vi "Lab Panel V5.40.vi"() -> ()   [LabVIEW 2017] (continued)
                    n2206 = Multiply(x=w3869, y=w3863) -> (x*y=w3856:dbl)
                    n2207 = Multiply(x=w3868, y=w3862) -> (x*y=w3854:dbl)
                    n2208 = Multiply(x=w3867, y=w3861) -> (x*y=w3853:dbl)
                    n2209 = Multiply(x=w3866, y=w3860) -> (x*y=w3852:dbl)
                    n2210 = local read "SIG LAB02-1"() -> (w3859:T2)
                    n2211 = local read "SIG LAB02-2"() -> (w3855:T2)
                    n2212 = Bundle By Name(cluster=w3859, "AMPS"=w3858, "VOLTS"=w3857, "PF"=w3856) -> (w3851:T2)
                    n2213 = Bundle By Name(cluster=w3855, "AMPS"=w3854, "VOLTS"=w3853, "PF"=w3852) -> (w3850:T2)
                    n2214 = global write "Global display 1.vi" "SIG LAB02-1"(w3851) -> ()
                    n2215 = local write "SIG LAB02-2"(w3850) -> ()
                    n2216 = global write "Global display 1.vi" "SIG LAB02-2"(w3850) -> ()
                    n2217 = local write "SIG LAB02-1"(w3851) -> ()
                  }
                  frame #4 {
                    n2218 = Unbundle By Name(w3903) -> ("OFF amps"=w3899:dbl, "VOLTS"=w3898:dbl, "PF"=w3897:dbl, "OFF amps"=w3896:dbl, "VOLTS"=w3895:dbl, "PF"=w3894:dbl)
                    n2219 = case shown="True" w3902 {
                      tunnel: [w3904 w3905] -> w3900
                      tunnel: w3901 -> [_ w3905]
                      frame False {
                        n2220 = local read "CAL LAB03"() -> (w3904:T15)
                      }
                      frame True {
                      }
                    }
                    n2221 = Unbundle By Name(w3900) -> ("1  (A) cal"=w3893:dbl, "1 (V) cal"=w3892:dbl, "1 (PF) cal"=w3891:dbl, "2 (A) cal"=w3890:dbl, "2 (V) cal"=w3889:dbl, "2 (PF) cal"=w3888:dbl)  [unwired: 4 out]
                    n2222 = Multiply(x=w3899, y=w3893) -> (x*y=w3886:dbl)
                    n2223 = Multiply(x=w3898, y=w3892) -> (x*y=w3880:dbl)
                    n2224 = Multiply(x=w3897, y=w3891) -> (x*y=w3885:dbl)
                    n2225 = Multiply(x=w3896, y=w3890) -> (x*y=w3883:dbl)
                    n2226 = Multiply(x=w3895, y=w3889) -> (x*y=w3882:dbl)
                    n2227 = Multiply(x=w3894, y=w3888) -> (x*y=w3881:dbl)
                    n2228 = local read "SIG LAB03-1"() -> (w3887:T2)
                    n2229 = local read "SIG LAB03-2"() -> (w3884:T2)
                    n2230 = Bundle By Name(cluster=w3887, "AMPS"=w3886, "VOLTS"=w3880, "PF"=w3885) -> (w3879:T2)
                    n2231 = Bundle By Name(cluster=w3884, "AMPS"=w3883, "VOLTS"=w3882, "PF"=w3881) -> (w3878:T2)
                    n2232 = global write "Global display 1.vi" "SIG LAB03-1"(w3879) -> ()
                    n2233 = global write "Global display 1.vi" "SIG LAB03-2"(w3878) -> ()
                    n2234 = local write "SIG LAB03-2"(w3878) -> ()
                    n2235 = local write "SIG LAB03-1"(w3879) -> ()
                  }
                  frame #5 {
                    n2236 = case shown="False" w3930 {
                      tunnel: [w3932 w3933] -> w3928
                      tunnel: w3929 -> [_ w3933]
                      frame False {
                        n2237 = local read "CAL LAB04"() -> (w3932:T15)
                      }
                      frame True {
                      }
                    }
                    n2238 = Unbundle By Name(w3931) -> ("OFF amps"=w3927:dbl, "VOLTS"=w3926:dbl, "PF"=w3925:dbl, "OFF amps"=w3924:dbl, "VOLTS"=w3923:dbl, "PF"=w3922:dbl)
                    n2239 = Unbundle By Name(w3928) -> ("1  (A) cal"=w3921:dbl, "1 (V) cal"=w3920:dbl, "1 (PF) cal"=w3919:dbl, "2 (A) cal"=w3918:dbl, "2 (V) cal"=w3917:dbl, "2 (PF) cal"=w3916:dbl)  [unwired: 4 out]
                    n2240 = Multiply(x=w3927, y=w3921) -> (x*y=w3914:dbl)
                    n2241 = Multiply(x=w3926, y=w3920) -> (x*y=w3913:dbl)
                    n2242 = Multiply(x=w3925, y=w3919) -> (x*y=w3912:dbl)
                    n2243 = Multiply(x=w3924, y=w3918) -> (x*y=w3910:dbl)
                    n2244 = Multiply(x=w3923, y=w3917) -> (x*y=w3909:dbl)
                    n2245 = Multiply(x=w3922, y=w3916) -> (x*y=w3908:dbl)
                    n2246 = local read "SIG LAB04-1"() -> (w3915:T2)
                    n2247 = local read "SIG LAB04-2"() -> (w3911:T2)
                    n2248 = Bundle By Name(cluster=w3915, "AMPS"=w3914, "VOLTS"=w3913, "PF"=w3912) -> (w3907:T2)
                    n2249 = Bundle By Name(cluster=w3911, "AMPS"=w3910, "VOLTS"=w3909, "PF"=w3908) -> (w3906:T2)
                    n2250 = global write "Global display 1.vi" "SIG LAB04-2"(w3906) -> ()
                    n2251 = global write "Global display 1.vi" "SIG LAB04-1"(w3907) -> ()
                    n2252 = local write "SIG LAB04-2"(w3906) -> ()
                    n2253 = local write "SIG LAB04-1"(w3907) -> ()
                  }
                  frame #6 {
                    n2254 = Unbundle By Name(w3959) -> ("OFF amps"=w3955:dbl, "VOLTS"=w3936:dbl, "PF"=w3954:dbl, "OFF amps"=w3953:dbl, "VOLTS"=w3952:dbl, "PF"=w3951:dbl)
                    n2255 = case shown="False" w3958 {
                      tunnel: [w3960 w3961] -> w3956
                      tunnel: w3957 -> [_ w3961]
                      frame False {
                        n2256 = local read "CAL LAB05"() -> (w3960:T15)
                      }
                      frame True {
                      }
                    }
                    n2257 = Unbundle By Name(w3956) -> ("1  (A) cal"=w3950:dbl, "1 (V) cal"=w3949:dbl, "1 (PF) cal"=w3948:dbl, "2 (A) cal"=w3947:dbl, "2 (V) cal"=w3946:dbl, "2 (PF) cal"=w3945:dbl)  [unwired: 4 out]
                    n2258 = Multiply(x=w3955, y=w3950) -> (x*y=w3943:dbl)
                    n2259 = Multiply(x=w3936, y=w3949) -> (x*y=w3942:dbl)
                    n2260 = Multiply(x=w3954, y=w3948) -> (x*y=w3941:dbl)
                    n2261 = Multiply(x=w3953, y=w3947) -> (x*y=w3939:dbl)
                    n2262 = Multiply(x=w3952, y=w3946) -> (x*y=w3938:dbl)
                    n2263 = Multiply(x=w3951, y=w3945) -> (x*y=w3937:dbl)
                    n2264 = local read "SIG LAB05-1"() -> (w3944:T2)
                    n2265 = local read "SIG LAB05-2"() -> (w3940:T2)
                    n2266 = Bundle By Name(cluster=w3944, "AMPS"=w3943, "VOLTS"=w3942, "PF"=w3941) -> (w3935:T2)
                    n2267 = Bundle By Name(cluster=w3940, "AMPS"=w3939, "VOLTS"=w3938, "PF"=w3937) -> (w3934:T2)
                    n2268 = global write "Global display 1.vi" "SIG LAB05-1"(w3935) -> ()
                    n2269 = global write "Global display 1.vi" "SIG LAB05-2"(w3934) -> ()
                    n2270 = local write "SIG LAB05-2"(w3934) -> ()
                    n2271 = local write "SIG LAB05-1"(w3935) -> ()
                  }
                  frame #7 {
                    n2272 = case shown="False" w3962 {
                      tunnel: w3964 -> [w3969 _]
                      tunnel: w3963 -> [w3968 _]
                      frame False {
                        # "update ambient referance temperature"
                        n2273 = case shown="True" w3969 {
                          tunnel: [w3971 100.0] -> w3970
                          frame False {
                            n2274 = local read "TEMP REF cal"() -> (w3971:dbl)
                          }
                          frame True {
                          }
                        }
                        n2275 = disable-structure shown="Disabled" {
                          frame Disabled {
                            n2276 = local read "Temp read loop"() -> ()  [unwired: 1 out]
                          }
                          frame Enabled {
                          }
                        }
                        n2277 = Multiply(x=w3970, y=w3968) -> (x*y=w3967:dbl)
                        n2278 = Subtract(x=w3967, y=272) -> (x-y=w3965:dbl)
                        "Amb Tp" <- w3965
                        n2279 = local write "Ref deg C"(w3965) -> ()
                        "deg C (volts)" <- w3968
                      }
                      frame True {
                      }
                    }
                  }
                }
              }
            }
          }
          frame #14 {
            # "save test data to file during testing"
            n2280 = local read "on loops"() -> (w3992:dbl)
            n2281 = Get Date/Time In Seconds() -> (seconds since 1Jan1904=w3973:timestamp)
            "File Time Stamp" <- w3973
            n2282 = local read "jig cycle"() -> (w3989:dbl)
            n2283 = Format Date/Time String(time format string (%c)="%H:%M%:%S", seconds (now)=w3973) -> (date/time string=w3977:string)  [unwired: 1 in]
            n2284 = Add(x=w3992, y=4) -> (x+y=w3990:dbl)
            n2285 = Build Array(w3977) -> (w3976:string[])
            n2286 = Equal?(x=w3989, y=3) -> (x = y?=w3975:bool)
            n2287 = Equal?(x=w3989, y=w3990) -> (x = y?=w3974:bool)
            n2288 = stacked-sequence {
              tunnel: w3988 -> [w3998 _ _ _ _ _ _ _ _ _]
              tunnel: w3987 -> [_ w4074 _ _ _ _ _ _ _ _]
              tunnel: w3986 -> [_ _ w4154 _ _ _ _ _ _ _]
              tunnel: w3985 -> [_ _ _ w4234 _ _ _ _ _ _]
              tunnel: w3984 -> [_ _ _ _ w4314 _ _ _ _ _]
              tunnel: w3983 -> [_ _ _ _ _ w4394 _ _ _ _]
              tunnel: w3982 -> [_ _ _ _ _ _ w4474 _ _ _]
              tunnel: w3981 -> [_ _ _ _ _ _ _ w4554 _ _]
              tunnel: w3980 -> [_ _ _ _ _ _ _ _ w4634 _]
              tunnel: w3979 -> [_ _ _ _ _ _ _ _ _ w4714]
              tunnel: w3976 -> [w3997 w4078 w4158 w4238 w4318 w4398 w4478 w4558 w4638 w4718]
              tunnel: w3975 -> [w3996 w4077 w4157 w4237 w4317 w4397 w4477 w4557 w4637 w4717]
              tunnel: w3974 -> [w3995 w4076 w4156 w4236 w4316 w4396 w4476 w4556 w4636 w4716]
              tunnel: w3973 -> [w3994 w4075 w4155 w4235 w4315 w4395 w4475 w4555 w4635 w4715]
              frame #0 {
                n2289 = case shown="True" w3998 {
                  tunnel: w3997 -> [_ w4003]
                  tunnel: w3996 -> [_ w4002]
                  tunnel: w3995 -> [_ w4000]
                  tunnel: w3994 -> [_ w3999]
                  frame False {
                  }
                  frame True {
                    n2290 = local read "SIG LAB01-1"() -> (w4005:T2)
                    n2291 = local read "ON L01-1"() -> (w4001:cluster{"amps":dbl, "volts":dbl, "pf":dbl})
                    n2292 = local read "DISP LAB01-1"() -> (w4004:T4)
                    n2293 = Unbundle(w4005) -> ("AMPS"=w4011:dbl, "VOLTS"=w4009:dbl, "PF"=w4008:dbl, "Tmp Live"=w4007:dbl, "Tmp Neut"=w4010:dbl)
                    n2294 = Unbundle(w4004) -> ("CYCLE"=w4006:dbl)  [unwired: 2 out]
                    n2295 = stacked-sequence {
                      tunnel: w4011 -> [w4015 w4034]
                      tunnel: w4010 -> [_ w4033]
                      tunnel: w4009 -> [w4014 w4032]
                      tunnel: w4008 -> [w4013 w4031]
                      tunnel: w4007 -> [_ w4030]
                      tunnel: w4006 -> [_ w4029]
                      tunnel: w4003 -> [_ w4028]
                      tunnel: w4002 -> [w4016 _]
                      tunnel: w4001 -> [w4012 w4026]
                      tunnel: w4000 -> [_ w4027]
                      tunnel: w3999 -> [_ w4022]
                      frame #0 {
                        n2296 = case shown="True" w4016 {
                          tunnel: w4015 -> [_ w4021]
                          tunnel: w4014 -> [_ w4020]
                          tunnel: w4013 -> [_ w4019]
                          tunnel: w4012 -> [_ w4017]
                          frame False {
                          }
                          frame True {
                            n2297 = Bundle(cluster=w4017, "amps"=w4021, "volts"=w4020, "pf"=w4019) -> (w4018:cluster{"amps":dbl, "volts":dbl, "pf":dbl})
                            n2298 = local write "ON L01-1"(w4018) -> ()
                          }
                        }
                      }
                      frame #1 {
                        n2299 = Unbundle(w4026) -> ("amps"=w4025:dbl, "volts"=w4024:dbl, "pf"=w4023:dbl)
                        n2300 = case shown="True" w4027 {
                          tunnel: w4034 -> [_ w4035]
                          tunnel: w4033 -> [_ w4073]
                          tunnel: w4032 -> [_ _]
                          tunnel: w4031 -> [_ _]
                          tunnel: w4030 -> [_ w4072]
                          tunnel: w4029 -> [_ w4071]
                          tunnel: w4028 -> [_ w4039]
                          tunnel: w4025 -> [_ w4036]
                          tunnel: w4024 -> [_ w4068]
                          tunnel: w4023 -> [_ w4067]
                          tunnel: w4022 -> [_ w4037]
                          frame False {
                          }
                          frame True {
                            n2301 = local read "TDMS LAB01-1"() -> (w4070:refnum<k34>)
                            n2302 = Build Array(w4068) -> (w4064:dbl[])
                            n2303 = Build Array(w4067) -> (w4063:dbl[])
                            n2304 = Build Array(w4072) -> (w4062:dbl[])
                            n2305 = Build Array(w4073) -> (w4061:dbl[])
                            n2306 = Build Array(w4036) -> (w4066:dbl[])
                            n2307 = Build Array(w4035) -> (w4065:dbl[])
                            n2308 = Build Array(w4071) -> (w4060:dbl[])
                            n2309 = Build Array("AMPS ON", "AMPS OFF", "VOLTS", "PF", "TEMP Live", "TEMP Neut", "CYCLE") -> (w4044:string[])
                            n2310 = Bundle By Name("Y"=w4066, "t0"=w4037) -> (w4059:waveform(dbl))  [unwired: 1 in]
                            n2311 = Bundle By Name("Y"=w4065, "t0"=w4037) -> (w4058:waveform(dbl))  [unwired: 1 in]
                            n2312 = Bundle By Name("Y"=w4064, "t0"=w4037) -> (w4057:waveform(dbl))  [unwired: 1 in]
                            n2313 = Bundle By Name("Y"=w4063, "t0"=w4037) -> (w4056:waveform(dbl))  [unwired: 1 in]
                            n2314 = Bundle By Name("Y"=w4062, "t0"=w4037) -> (w4055:waveform(dbl))  [unwired: 1 in]
                            n2315 = Bundle By Name("Y"=w4061, "t0"=w4037) -> (w4054:waveform(dbl))  [unwired: 1 in]
                            n2316 = Bundle By Name("Y"=w4060, "t0"=w4037) -> (w4053:waveform(dbl))  [unwired: 1 in]
                            n2317 = Build Array(w4059, w4058, w4057, w4056, w4055, w4054, w4053) -> (w4052:waveform(dbl)[])
                            n2318 = TDMS Write(0:w4070, 5:"TEST VALUES", 7:w4044, 9:w4052) -> (4:w4043:refnum<k34>, 6:w4042:string, 15:w4041:errorcluster)  [unwired: 2 in, 1 out]
                            n2319 = TDMS Write(0:w4043, 5:w4042, 7:"TIME", 9:w4039, 11:w4041) -> (15:w4038:errorcluster)  [unwired: 1 in, 3 out]
                            n2320 = local write "data file error"(w4038) -> ()
                          }
                        }
                      }
                    }
                  }
                }
              }
              frame #1 {
                n2321 = case shown="True" w4074 {
                  tunnel: w4078 -> [_ w4083]
                  tunnel: w4077 -> [_ w4082]
                  tunnel: w4076 -> [_ w4080]
                  tunnel: w4075 -> [_ w4079]
                  frame False {
                  }
                  frame True {
                    n2322 = local read "DISP LAB01-2"() -> (w4084:T4)
                    n2323 = local read "SIG LAB01-2"() -> (w4085:T2)
                    n2324 = local read "ON L01-2"() -> (w4081:cluster{"amps":dbl, "volts":dbl, "pf":dbl})
                    n2325 = Unbundle(w4085) -> ("AMPS"=w4091:dbl, "VOLTS"=w4089:dbl, "PF"=w4088:dbl, "Tmp Live"=w4087:dbl, "Tmp Neut"=w4090:dbl)
                    n2326 = Unbundle(w4084) -> ("CYCLE"=w4086:dbl)  [unwired: 2 out]
                    n2327 = stacked-sequence {
                      tunnel: w4091 -> [w4095 w4114]
                      tunnel: w4090 -> [_ w4113]
                      tunnel: w4089 -> [w4094 w4112]
                      tunnel: w4088 -> [w4093 w4111]
                      tunnel: w4087 -> [_ w4110]
                      tunnel: w4086 -> [_ w4109]
                      tunnel: w4083 -> [_ w4108]
                      tunnel: w4082 -> [w4096 _]
                      tunnel: w4081 -> [w4092 w4106]
                      tunnel: w4080 -> [_ w4107]
                      tunnel: w4079 -> [_ w4102]
                      frame #0 {
                        n2328 = case shown="True" w4096 {
                          tunnel: w4095 -> [_ w4101]
                          tunnel: w4094 -> [_ w4100]
                          tunnel: w4093 -> [_ w4099]
                          tunnel: w4092 -> [_ w4097]
                          frame False {
                          }
                          frame True {
                            n2329 = Bundle(cluster=w4097, "amps"=w4101, "volts"=w4100, "pf"=w4099) -> (w4098:cluster{"amps":dbl, "volts":dbl, "pf":dbl})
                            n2330 = local write "ON L01-2"(w4098) -> ()
                          }
                        }
                      }
                      frame #1 {
                        n2331 = Unbundle(w4106) -> ("amps"=w4105:dbl, "volts"=w4104:dbl, "pf"=w4103:dbl)
                        n2332 = case shown="True" w4107 {
                          tunnel: w4114 -> [_ w4146]
                          tunnel: w4113 -> [_ w4153]
                          tunnel: w4112 -> [_ _]
                          tunnel: w4111 -> [_ _]
                          tunnel: w4110 -> [_ w4152]
                          tunnel: w4109 -> [_ w4151]
                          tunnel: w4108 -> [_ w4116]
                          tunnel: w4105 -> [_ w4148]
                          tunnel: w4104 -> [_ w4147]
                          tunnel: w4103 -> [_ w4145]
                          tunnel: w4102 -> [_ w4137]
                          frame False {
                          }
                          frame True {
                            n2333 = local read "TDMS LAB01-2"() -> (w4150:refnum<k34>)
                            n2334 = Build Array(w4147) -> (w4142:dbl[])
                            n2335 = Build Array(w4145) -> (w4141:dbl[])
                            n2336 = Build Array(w4152) -> (w4140:dbl[])
                            n2337 = Build Array(w4153) -> (w4139:dbl[])
                            n2338 = Build Array(w4148) -> (w4144:dbl[])
                            n2339 = Build Array(w4146) -> (w4143:dbl[])
                            n2340 = Build Array(w4151) -> (w4138:dbl[])
                            n2341 = Build Array("AMPS ON", "AMPS OFF", "VOLTS", "PF", "TEMP Live", "TEMP Neut", "CYCLE") -> (w4121:string[])
                            n2342 = Bundle By Name("Y"=w4144, "t0"=w4137) -> (w4136:waveform(dbl))  [unwired: 1 in]
                            n2343 = Bundle By Name("Y"=w4143, "t0"=w4137) -> (w4135:waveform(dbl))  [unwired: 1 in]
                            n2344 = Bundle By Name("Y"=w4142, "t0"=w4137) -> (w4134:waveform(dbl))  [unwired: 1 in]
                            n2345 = Bundle By Name("Y"=w4141, "t0"=w4137) -> (w4133:waveform(dbl))  [unwired: 1 in]
                            n2346 = Bundle By Name("Y"=w4140, "t0"=w4137) -> (w4132:waveform(dbl))  [unwired: 1 in]
                            n2347 = Bundle By Name("Y"=w4139, "t0"=w4137) -> (w4131:waveform(dbl))  [unwired: 1 in]
                            n2348 = Bundle By Name("Y"=w4138, "t0"=w4137) -> (w4130:waveform(dbl))  [unwired: 1 in]
                            n2349 = Build Array(w4136, w4135, w4134, w4133, w4132, w4131, w4130) -> (w4129:waveform(dbl)[])
                            n2350 = TDMS Write(0:w4150, 5:"TEST VALUES", 7:w4121, 9:w4129) -> (4:w4120:refnum<k34>, 6:w4119:string, 15:w4118:errorcluster)  [unwired: 2 in, 1 out]
                            n2351 = TDMS Write(0:w4120, 5:w4119, 7:"TIME", 9:w4116, 11:w4118) -> (15:w4115:errorcluster)  [unwired: 1 in, 3 out]
                            n2352 = local write "data file error"(w4115) -> ()
                          }
                        }
                      }
                    }
                  }
                }
              }
              frame #2 {
                n2353 = case shown="True" w4154 {
                  tunnel: w4158 -> [_ w4163]
                  tunnel: w4157 -> [_ w4162]
                  tunnel: w4156 -> [_ w4160]
                  tunnel: w4155 -> [_ w4159]
                  frame False {
                  }
                  frame True {
                    n2354 = local read "DISP LAB02-1"() -> (w4164:T4)
                    n2355 = local read "SIG LAB02-1"() -> (w4165:T2)
                    n2356 = local read "ON L02-1"() -> (w4161:cluster{"amps":dbl, "volts":dbl, "pf":dbl})
                    n2357 = Unbundle(w4165) -> ("AMPS"=w4171:dbl, "VOLTS"=w4169:dbl, "PF"=w4168:dbl, "Tmp Live"=w4167:dbl, "Tmp Neut"=w4170:dbl)
                    n2358 = Unbundle(w4164) -> ("CYCLE"=w4166:dbl)  [unwired: 2 out]
                    n2359 = stacked-sequence {
                      tunnel: w4171 -> [w4175 w4194]
                      tunnel: w4170 -> [_ w4193]
                      tunnel: w4169 -> [w4174 w4192]
                      tunnel: w4168 -> [w4173 w4191]
                      tunnel: w4167 -> [_ w4190]
                      tunnel: w4166 -> [_ w4189]
                      tunnel: w4163 -> [_ w4188]
                      tunnel: w4162 -> [w4176 _]
                      tunnel: w4161 -> [w4172 w4186]
                      tunnel: w4160 -> [_ w4187]
                      tunnel: w4159 -> [_ w4182]
                      frame #0 {
                        n2360 = case shown="True" w4176 {
                          tunnel: w4175 -> [_ w4181]
                          tunnel: w4174 -> [_ w4180]
                          tunnel: w4173 -> [_ w4179]
                          tunnel: w4172 -> [_ w4177]
                          frame False {
                          }
                          frame True {
                            n2361 = Bundle(cluster=w4177, "amps"=w4181, "volts"=w4180, "pf"=w4179) -> (w4178:cluster{"amps":dbl, "volts":dbl, "pf":dbl})
                            n2362 = local write "ON L02-1"(w4178) -> ()
                          }
                        }
                      }
                      frame #1 {
                        n2363 = Unbundle(w4186) -> ("amps"=w4185:dbl, "volts"=w4184:dbl, "pf"=w4183:dbl)
                        n2364 = case shown="True" w4187 {
                          tunnel: w4194 -> [_ w4226]
                          tunnel: w4193 -> [_ w4233]
                          tunnel: w4192 -> [_ _]
                          tunnel: w4191 -> [_ _]
                          tunnel: w4190 -> [_ w4232]
                          tunnel: w4189 -> [_ w4231]
                          tunnel: w4188 -> [_ w4196]
                          tunnel: w4185 -> [_ w4228]
                          tunnel: w4184 -> [_ w4227]
                          tunnel: w4183 -> [_ w4225]
                          tunnel: w4182 -> [_ w4217]
                          frame False {
                          }
                          frame True {
                            n2365 = local read "TDMS LAB02-1"() -> (w4230:refnum<k34>)
                            n2366 = Build Array(w4227) -> (w4222:dbl[])
                            n2367 = Build Array(w4225) -> (w4221:dbl[])
                            n2368 = Build Array(w4232) -> (w4220:dbl[])
                            n2369 = Build Array(w4233) -> (w4219:dbl[])
                            n2370 = Build Array(w4228) -> (w4224:dbl[])
                            n2371 = Build Array(w4226) -> (w4223:dbl[])
                            n2372 = Build Array(w4231) -> (w4218:dbl[])
                            n2373 = Build Array("AMPS ON", "AMPS OFF", "VOLTS", "PF", "TEMP Live", "TEMP Neut", "CYCLE") -> (w4201:string[])
                            n2374 = Bundle By Name("Y"=w4224, "t0"=w4217) -> (w4216:waveform(dbl))  [unwired: 1 in]
                            n2375 = Bundle By Name("Y"=w4223, "t0"=w4217) -> (w4215:waveform(dbl))  [unwired: 1 in]
                            n2376 = Bundle By Name("Y"=w4222, "t0"=w4217) -> (w4214:waveform(dbl))  [unwired: 1 in]
                            n2377 = Bundle By Name("Y"=w4221, "t0"=w4217) -> (w4213:waveform(dbl))  [unwired: 1 in]
                            n2378 = Bundle By Name("Y"=w4220, "t0"=w4217) -> (w4212:waveform(dbl))  [unwired: 1 in]
                            n2379 = Bundle By Name("Y"=w4219, "t0"=w4217) -> (w4211:waveform(dbl))  [unwired: 1 in]
                            n2380 = Bundle By Name("Y"=w4218, "t0"=w4217) -> (w4210:waveform(dbl))  [unwired: 1 in]
                            n2381 = Build Array(w4216, w4215, w4214, w4213, w4212, w4211, w4210) -> (w4209:waveform(dbl)[])
                            n2382 = TDMS Write(0:w4230, 5:"TEST VALUES", 7:w4201, 9:w4209) -> (4:w4200:refnum<k34>, 6:w4199:string, 15:w4198:errorcluster)  [unwired: 2 in, 1 out]
                            n2383 = TDMS Write(0:w4200, 5:w4199, 7:"TIME", 9:w4196, 11:w4198) -> (15:w4195:errorcluster)  [unwired: 1 in, 3 out]
                            n2384 = local write "data file error"(w4195) -> ()
                          }
                        }
                      }
                    }
                  }
                }
              }
              frame #3 {
                n2385 = case shown="True" w4234 {
                  tunnel: w4238 -> [_ w4243]
                  tunnel: w4237 -> [_ w4242]
                  tunnel: w4236 -> [_ w4240]
                  tunnel: w4235 -> [_ w4239]
                  frame False {
                  }
                  frame True {
                    n2386 = local read "DISP LAB02-2"() -> (w4244:T4)
                    n2387 = local read "SIG LAB02-2"() -> (w4245:T2)
                    n2388 = local read "ON L02-2"() -> (w4241:cluster{"amps":dbl, "volts":dbl, "pf":dbl})
                    n2389 = Unbundle(w4245) -> ("AMPS"=w4251:dbl, "VOLTS"=w4249:dbl, "PF"=w4248:dbl, "Tmp Live"=w4247:dbl, "Tmp Neut"=w4250:dbl)
                    n2390 = Unbundle(w4244) -> ("CYCLE"=w4246:dbl)  [unwired: 2 out]
                    n2391 = stacked-sequence {
                      tunnel: w4251 -> [w4255 w4274]
                      tunnel: w4250 -> [_ w4273]
                      tunnel: w4249 -> [w4254 w4272]
                      tunnel: w4248 -> [w4253 w4271]
                      tunnel: w4247 -> [_ w4270]
                      tunnel: w4246 -> [_ w4269]
                      tunnel: w4243 -> [_ w4268]
                      tunnel: w4242 -> [w4256 _]
                      tunnel: w4241 -> [w4252 w4266]
                      tunnel: w4240 -> [_ w4267]
                      tunnel: w4239 -> [_ w4262]
                      frame #0 {
                        n2392 = case shown="True" w4256 {
                          tunnel: w4255 -> [_ w4261]
                          tunnel: w4254 -> [_ w4260]
                          tunnel: w4253 -> [_ w4259]
                          tunnel: w4252 -> [_ w4257]
                          frame False {
                          }
                          frame True {
                            n2393 = Bundle(cluster=w4257, "amps"=w4261, "volts"=w4260, "pf"=w4259) -> (w4258:cluster{"amps":dbl, "volts":dbl, "pf":dbl})
                            n2394 = local write "ON L02-2"(w4258) -> ()
                          }
                        }
                      }
                      frame #1 {
                        n2395 = Unbundle(w4266) -> ("amps"=w4265:dbl, "volts"=w4264:dbl, "pf"=w4263:dbl)
                        n2396 = case shown="True" w4267 {
                          tunnel: w4274 -> [_ w4306]
                          tunnel: w4273 -> [_ w4313]
                          tunnel: w4272 -> [_ _]
                          tunnel: w4271 -> [_ _]
                          tunnel: w4270 -> [_ w4312]
                          tunnel: w4269 -> [_ w4311]
                          tunnel: w4268 -> [_ w4276]
                          tunnel: w4265 -> [_ w4308]
                          tunnel: w4264 -> [_ w4307]
                          tunnel: w4263 -> [_ w4305]
                          tunnel: w4262 -> [_ w4297]
                          frame False {
                          }
                          frame True {
                            n2397 = local read "TDMS LAB02-2"() -> (w4310:refnum<k34>)
                            n2398 = Build Array(w4307) -> (w4302:dbl[])
                            n2399 = Build Array(w4305) -> (w4301:dbl[])
                            n2400 = Build Array(w4312) -> (w4300:dbl[])
                            n2401 = Build Array(w4313) -> (w4299:dbl[])
                            n2402 = Build Array(w4308) -> (w4304:dbl[])
                            n2403 = Build Array(w4306) -> (w4303:dbl[])
                            n2404 = Build Array(w4311) -> (w4298:dbl[])
                            n2405 = Build Array("AMPS ON", "AMPS OFF", "VOLTS", "PF", "TEMP Live", "TEMP Neut", "CYCLE") -> (w4281:string[])
                            n2406 = Bundle By Name("Y"=w4304, "t0"=w4297) -> (w4296:waveform(dbl))  [unwired: 1 in]
                            n2407 = Bundle By Name("Y"=w4303, "t0"=w4297) -> (w4295:waveform(dbl))  [unwired: 1 in]
                            n2408 = Bundle By Name("Y"=w4302, "t0"=w4297) -> (w4294:waveform(dbl))  [unwired: 1 in]
                            n2409 = Bundle By Name("Y"=w4301, "t0"=w4297) -> (w4293:waveform(dbl))  [unwired: 1 in]
                            n2410 = Bundle By Name("Y"=w4300, "t0"=w4297) -> (w4292:waveform(dbl))  [unwired: 1 in]
                            n2411 = Bundle By Name("Y"=w4299, "t0"=w4297) -> (w4291:waveform(dbl))  [unwired: 1 in]
                            n2412 = Bundle By Name("Y"=w4298, "t0"=w4297) -> (w4290:waveform(dbl))  [unwired: 1 in]
                            n2413 = Build Array(w4296, w4295, w4294, w4293, w4292, w4291, w4290) -> (w4289:waveform(dbl)[])
                            n2414 = TDMS Write(0:w4310, 5:"TEST VALUES", 7:w4281, 9:w4289) -> (4:w4280:refnum<k34>, 6:w4279:string, 15:w4278:errorcluster)  [unwired: 2 in, 1 out]
                            n2415 = TDMS Write(0:w4280, 5:w4279, 7:"TIME", 9:w4276, 11:w4278) -> (15:w4275:errorcluster)  [unwired: 1 in, 3 out]
                            n2416 = local write "data file error"(w4275) -> ()
                          }
                        }
                      }
                    }
                  }
                }
              }
              frame #4 {
                n2417 = case shown="True" w4314 {
                  tunnel: w4318 -> [_ w4323]
                  tunnel: w4317 -> [_ w4322]
                  tunnel: w4316 -> [_ w4320]
                  tunnel: w4315 -> [_ w4319]
                  frame False {
                  }
                  frame True {
                    n2418 = local read "DISP LAB03-1"() -> (w4324:T4)
                    n2419 = local read "SIG LAB03-1"() -> (w4325:T2)
                    n2420 = local read "ON L03-1"() -> (w4321:cluster{"amps":dbl, "volts":dbl, "pf":dbl})
                    n2421 = Unbundle(w4325) -> ("AMPS"=w4331:dbl, "VOLTS"=w4329:dbl, "PF"=w4328:dbl, "Tmp Live"=w4327:dbl, "Tmp Neut"=w4330:dbl)
                    n2422 = Unbundle(w4324) -> ("CYCLE"=w4326:dbl)  [unwired: 2 out]
                    n2423 = stacked-sequence {
                      tunnel: w4331 -> [w4335 w4354]
                      tunnel: w4330 -> [_ w4353]
                      tunnel: w4329 -> [w4334 w4352]
                      tunnel: w4328 -> [w4333 w4351]
                      tunnel: w4327 -> [_ w4350]
                      tunnel: w4326 -> [_ w4349]
                      tunnel: w4323 -> [_ w4348]
                      tunnel: w4322 -> [w4336 _]
                      tunnel: w4321 -> [w4332 w4346]
                      tunnel: w4320 -> [_ w4347]
                      tunnel: w4319 -> [_ w4342]
                      frame #0 {
                        n2424 = case shown="True" w4336 {
                          tunnel: w4335 -> [_ w4341]
                          tunnel: w4334 -> [_ w4340]
                          tunnel: w4333 -> [_ w4339]
                          tunnel: w4332 -> [_ w4337]
                          frame False {
                          }
                          frame True {
                            n2425 = Bundle(cluster=w4337, "amps"=w4341, "volts"=w4340, "pf"=w4339) -> (w4338:cluster{"amps":dbl, "volts":dbl, "pf":dbl})
                            n2426 = local write "ON L03-1"(w4338) -> ()
                          }
                        }
                      }
                      frame #1 {
                        n2427 = Unbundle(w4346) -> ("amps"=w4345:dbl, "volts"=w4344:dbl, "pf"=w4343:dbl)
                        n2428 = case shown="True" w4347 {
                          tunnel: w4354 -> [_ w4386]
                          tunnel: w4353 -> [_ w4393]
                          tunnel: w4352 -> [_ _]
                          tunnel: w4351 -> [_ _]
                          tunnel: w4350 -> [_ w4392]
                          tunnel: w4349 -> [_ w4391]
                          tunnel: w4348 -> [_ w4356]
                          tunnel: w4345 -> [_ w4388]
                          tunnel: w4344 -> [_ w4387]
                          tunnel: w4343 -> [_ w4385]
                          tunnel: w4342 -> [_ w4377]
                          frame False {
                          }
                          frame True {
                            n2429 = local read "TDMS LAB03-1"() -> (w4390:refnum<k34>)
                            n2430 = Build Array(w4387) -> (w4382:dbl[])
                            n2431 = Build Array(w4385) -> (w4381:dbl[])
                            n2432 = Build Array(w4392) -> (w4380:dbl[])
                            n2433 = Build Array(w4393) -> (w4379:dbl[])
                            n2434 = Build Array(w4388) -> (w4384:dbl[])
                            n2435 = Build Array(w4386) -> (w4383:dbl[])
                            n2436 = Build Array(w4391) -> (w4378:dbl[])
                            n2437 = Build Array("AMPS ON", "AMPS OFF", "VOLTS", "PF", "TEMP Live", "TEMP Neut", "CYCLE") -> (w4361:string[])
                            n2438 = Bundle By Name("Y"=w4384, "t0"=w4377) -> (w4376:waveform(dbl))  [unwired: 1 in]
                            n2439 = Bundle By Name("Y"=w4383, "t0"=w4377) -> (w4375:waveform(dbl))  [unwired: 1 in]
                            n2440 = Bundle By Name("Y"=w4382, "t0"=w4377) -> (w4374:waveform(dbl))  [unwired: 1 in]
                            n2441 = Bundle By Name("Y"=w4381, "t0"=w4377) -> (w4373:waveform(dbl))  [unwired: 1 in]
                            n2442 = Bundle By Name("Y"=w4380, "t0"=w4377) -> (w4372:waveform(dbl))  [unwired: 1 in]
                            n2443 = Bundle By Name("Y"=w4379, "t0"=w4377) -> (w4371:waveform(dbl))  [unwired: 1 in]
                            n2444 = Bundle By Name("Y"=w4378, "t0"=w4377) -> (w4370:waveform(dbl))  [unwired: 1 in]
                            n2445 = Build Array(w4376, w4375, w4374, w4373, w4372, w4371, w4370) -> (w4369:waveform(dbl)[])
                            n2446 = TDMS Write(0:w4390, 5:"TEST VALUES", 7:w4361, 9:w4369) -> (4:w4360:refnum<k34>, 6:w4359:string, 15:w4358:errorcluster)  [unwired: 2 in, 1 out]
                            n2447 = TDMS Write(0:w4360, 5:w4359, 7:"TIME", 9:w4356, 11:w4358) -> (15:w4355:errorcluster)  [unwired: 1 in, 3 out]
                            n2448 = local write "data file error"(w4355) -> ()
                          }
                        }
                      }
                    }
                  }
                }
              }
              frame #5 {
                n2449 = case shown="True" w4394 {
                  tunnel: w4398 -> [_ w4403]
                  tunnel: w4397 -> [_ w4402]
                  tunnel: w4396 -> [_ w4400]
                  tunnel: w4395 -> [_ w4399]
                  frame False {
                  }
                  frame True {
                    n2450 = local read "DISP LAB03-2"() -> (w4404:T4)
                    n2451 = local read "SIG LAB03-2"() -> (w4405:T2)
                    n2452 = local read "ON L03-2"() -> (w4401:cluster{"amps":dbl, "volts":dbl, "pf":dbl})
                    n2453 = Unbundle(w4405) -> ("AMPS"=w4411:dbl, "VOLTS"=w4409:dbl, "PF"=w4408:dbl, "Tmp Live"=w4407:dbl, "Tmp Neut"=w4410:dbl)
                    n2454 = Unbundle(w4404) -> ("CYCLE"=w4406:dbl)  [unwired: 2 out]
                    n2455 = stacked-sequence {
                      tunnel: w4411 -> [w4415 w4434]
                      tunnel: w4410 -> [_ w4433]
                      tunnel: w4409 -> [w4414 w4432]
                      tunnel: w4408 -> [w4413 w4431]
                      tunnel: w4407 -> [_ w4430]
                      tunnel: w4406 -> [_ w4429]
                      tunnel: w4403 -> [_ w4428]
                      tunnel: w4402 -> [w4416 _]
                      tunnel: w4401 -> [w4412 w4426]
                      tunnel: w4400 -> [_ w4427]
                      tunnel: w4399 -> [_ w4422]
                      frame #0 {
                        n2456 = case shown="True" w4416 {
                          tunnel: w4415 -> [_ w4421]
                          tunnel: w4414 -> [_ w4420]
                          tunnel: w4413 -> [_ w4419]
                          tunnel: w4412 -> [_ w4417]
                          frame False {
                          }
                          frame True {
                            n2457 = Bundle(cluster=w4417, "amps"=w4421, "volts"=w4420, "pf"=w4419) -> (w4418:cluster{"amps":dbl, "volts":dbl, "pf":dbl})
                            n2458 = local write "ON L03-2"(w4418) -> ()
                          }
                        }
                      }
                      frame #1 {
                        n2459 = Unbundle(w4426) -> ("amps"=w4425:dbl, "volts"=w4424:dbl, "pf"=w4423:dbl)
                        n2460 = case shown="True" w4427 {
                          tunnel: w4434 -> [_ w4466]
                          tunnel: w4433 -> [_ w4473]
                          tunnel: w4432 -> [_ _]
                          tunnel: w4431 -> [_ _]
                          tunnel: w4430 -> [_ w4472]
                          tunnel: w4429 -> [_ w4471]
                          tunnel: w4428 -> [_ w4436]
                          tunnel: w4425 -> [_ w4468]
                          tunnel: w4424 -> [_ w4467]
                          tunnel: w4423 -> [_ w4465]
                          tunnel: w4422 -> [_ w4457]
                          frame False {
                          }
                          frame True {
                            n2461 = local read "TDMS LAB03-2"() -> (w4470:refnum<k34>)
                            n2462 = Build Array(w4467) -> (w4462:dbl[])
                            n2463 = Build Array(w4465) -> (w4461:dbl[])
                            n2464 = Build Array(w4472) -> (w4460:dbl[])
                            n2465 = Build Array(w4473) -> (w4459:dbl[])
                            n2466 = Build Array(w4468) -> (w4464:dbl[])
                            n2467 = Build Array(w4466) -> (w4463:dbl[])
                            n2468 = Build Array(w4471) -> (w4458:dbl[])
                            n2469 = Build Array("AMPS ON", "AMPS OFF", "VOLTS", "PF", "TEMP Live", "TEMP Neut", "CYCLE") -> (w4441:string[])
                            n2470 = Bundle By Name("Y"=w4464, "t0"=w4457) -> (w4456:waveform(dbl))  [unwired: 1 in]
                            n2471 = Bundle By Name("Y"=w4463, "t0"=w4457) -> (w4455:waveform(dbl))  [unwired: 1 in]
                            n2472 = Bundle By Name("Y"=w4462, "t0"=w4457) -> (w4454:waveform(dbl))  [unwired: 1 in]
                            n2473 = Bundle By Name("Y"=w4461, "t0"=w4457) -> (w4453:waveform(dbl))  [unwired: 1 in]
                            n2474 = Bundle By Name("Y"=w4460, "t0"=w4457) -> (w4452:waveform(dbl))  [unwired: 1 in]
                            n2475 = Bundle By Name("Y"=w4459, "t0"=w4457) -> (w4451:waveform(dbl))  [unwired: 1 in]
                            n2476 = Bundle By Name("Y"=w4458, "t0"=w4457) -> (w4450:waveform(dbl))  [unwired: 1 in]
                            n2477 = Build Array(w4456, w4455, w4454, w4453, w4452, w4451, w4450) -> (w4449:waveform(dbl)[])
                            n2478 = TDMS Write(0:w4470, 5:"TEST VALUES", 7:w4441, 9:w4449) -> (4:w4440:refnum<k34>, 6:w4439:string, 15:w4438:errorcluster)  [unwired: 2 in, 1 out]
                            n2479 = TDMS Write(0:w4440, 5:w4439, 7:"TIME", 9:w4436, 11:w4438) -> (15:w4435:errorcluster)  [unwired: 1 in, 3 out]
                            n2480 = local write "data file error"(w4435) -> ()
                          }
                        }
                      }
                    }
                  }
                }
              }
              frame #6 {
                n2481 = case shown="True" w4474 {
                  tunnel: w4478 -> [_ w4483]
                  tunnel: w4477 -> [_ w4482]
                  tunnel: w4476 -> [_ w4480]
                  tunnel: w4475 -> [_ w4479]
                  frame False {
                  }
                  frame True {
                    n2482 = local read "DISP LAB04-1"() -> (w4484:T4)
                    n2483 = local read "SIG LAB04-1"() -> (w4485:T2)
                    n2484 = local read "ON L04-1"() -> (w4481:cluster{"amps":dbl, "volts":dbl, "pf":dbl})
                    n2485 = Unbundle(w4485) -> ("AMPS"=w4491:dbl, "VOLTS"=w4489:dbl, "PF"=w4488:dbl, "Tmp Live"=w4487:dbl, "Tmp Neut"=w4490:dbl)
                    n2486 = Unbundle(w4484) -> ("CYCLE"=w4486:dbl)  [unwired: 2 out]
                    n2487 = stacked-sequence {
                      tunnel: w4491 -> [w4495 w4514]
                      tunnel: w4490 -> [_ w4513]
                      tunnel: w4489 -> [w4494 w4512]
                      tunnel: w4488 -> [w4493 w4511]
                      tunnel: w4487 -> [_ w4510]
                      tunnel: w4486 -> [_ w4509]
                      tunnel: w4483 -> [_ w4508]
                      tunnel: w4482 -> [w4496 _]
                      tunnel: w4481 -> [w4492 w4506]
                      tunnel: w4480 -> [_ w4507]
                      tunnel: w4479 -> [_ w4502]
                      frame #0 {
                        n2488 = case shown="True" w4496 {
                          tunnel: w4495 -> [_ w4501]
                          tunnel: w4494 -> [_ w4500]
                          tunnel: w4493 -> [_ w4499]
                          tunnel: w4492 -> [_ w4497]
                          frame False {
                          }
                          frame True {
                            n2489 = Bundle(cluster=w4497, "amps"=w4501, "volts"=w4500, "pf"=w4499) -> (w4498:cluster{"amps":dbl, "volts":dbl, "pf":dbl})
                            n2490 = local write "ON L04-1"(w4498) -> ()
                          }
                        }
                      }
                      frame #1 {
                        n2491 = Unbundle(w4506) -> ("amps"=w4505:dbl, "volts"=w4504:dbl, "pf"=w4503:dbl)
                        n2492 = case shown="True" w4507 {
                          tunnel: w4514 -> [_ w4546]
                          tunnel: w4513 -> [_ w4553]
                          tunnel: w4512 -> [_ _]
                          tunnel: w4511 -> [_ _]
                          tunnel: w4510 -> [_ w4552]
                          tunnel: w4509 -> [_ w4551]
                          tunnel: w4508 -> [_ w4516]
                          tunnel: w4505 -> [_ w4548]
                          tunnel: w4504 -> [_ w4547]
                          tunnel: w4503 -> [_ w4545]
                          tunnel: w4502 -> [_ w4537]
                          frame False {
                          }
                          frame True {
                            n2493 = local read "TDMS LAB04-1"() -> (w4550:refnum<k34>)
                            n2494 = Build Array(w4547) -> (w4542:dbl[])
                            n2495 = Build Array(w4545) -> (w4541:dbl[])
                            n2496 = Build Array(w4552) -> (w4540:dbl[])
                            n2497 = Build Array(w4553) -> (w4539:dbl[])
                            n2498 = Build Array(w4548) -> (w4544:dbl[])
                            n2499 = Build Array(w4546) -> (w4543:dbl[])
                            n2500 = Build Array(w4551) -> (w4538:dbl[])
                            n2501 = Build Array("AMPS ON", "AMPS OFF", "VOLTS", "PF", "TEMP Live", "TEMP Neut", "CYCLE") -> (w4521:string[])
                            n2502 = Bundle By Name("Y"=w4544, "t0"=w4537) -> (w4536:waveform(dbl))  [unwired: 1 in]
                            n2503 = Bundle By Name("Y"=w4543, "t0"=w4537) -> (w4535:waveform(dbl))  [unwired: 1 in]
                            n2504 = Bundle By Name("Y"=w4542, "t0"=w4537) -> (w4534:waveform(dbl))  [unwired: 1 in]
                            n2505 = Bundle By Name("Y"=w4541, "t0"=w4537) -> (w4533:waveform(dbl))  [unwired: 1 in]
                            n2506 = Bundle By Name("Y"=w4540, "t0"=w4537) -> (w4532:waveform(dbl))  [unwired: 1 in]
                            n2507 = Bundle By Name("Y"=w4539, "t0"=w4537) -> (w4531:waveform(dbl))  [unwired: 1 in]
                            n2508 = Bundle By Name("Y"=w4538, "t0"=w4537) -> (w4530:waveform(dbl))  [unwired: 1 in]
                            n2509 = Build Array(w4536, w4535, w4534, w4533, w4532, w4531, w4530) -> (w4529:waveform(dbl)[])
                            n2510 = TDMS Write(0:w4550, 5:"TEST VALUES", 7:w4521, 9:w4529) -> (4:w4520:refnum<k34>, 6:w4519:string, 15:w4518:errorcluster)  [unwired: 2 in, 1 out]
                            n2511 = TDMS Write(0:w4520, 5:w4519, 7:"TIME", 9:w4516, 11:w4518) -> (15:w4515:errorcluster)  [unwired: 1 in, 3 out]
                            n2512 = local write "data file error"(w4515) -> ()
                          }
                        }
                      }
                    }
                  }
                }
              }
              frame #7 {
                n2513 = case shown="True" w4554 {
                  tunnel: w4558 -> [_ w4563]
                  tunnel: w4557 -> [_ w4562]
                  tunnel: w4556 -> [_ w4560]
                  tunnel: w4555 -> [_ w4559]
                  frame False {
                  }
                  frame True {
                    n2514 = local read "DISP LAB04-2"() -> (w4564:T4)
                    n2515 = local read "SIG LAB04-2"() -> (w4565:T2)
                    n2516 = local read "ON L04-2"() -> (w4561:cluster{"amps":dbl, "volts":dbl, "pf":dbl})
                    n2517 = Unbundle(w4565) -> ("AMPS"=w4571:dbl, "VOLTS"=w4569:dbl, "PF"=w4568:dbl, "Tmp Live"=w4567:dbl, "Tmp Neut"=w4570:dbl)
                    n2518 = Unbundle(w4564) -> ("CYCLE"=w4566:dbl)  [unwired: 2 out]
                    n2519 = stacked-sequence {
                      tunnel: w4571 -> [w4575 w4594]
                      tunnel: w4570 -> [_ w4593]
                      tunnel: w4569 -> [w4574 w4592]
                      tunnel: w4568 -> [w4573 w4591]
                      tunnel: w4567 -> [_ w4590]
                      tunnel: w4566 -> [_ w4589]
                      tunnel: w4563 -> [_ w4588]
                      tunnel: w4562 -> [w4576 _]
                      tunnel: w4561 -> [w4572 w4586]
                      tunnel: w4560 -> [_ w4587]
                      tunnel: w4559 -> [_ w4582]
                      frame #0 {
                        n2520 = case shown="True" w4576 {
                          tunnel: w4575 -> [_ w4581]
                          tunnel: w4574 -> [_ w4580]
                          tunnel: w4573 -> [_ w4579]
                          tunnel: w4572 -> [_ w4577]
                          frame False {
                          }
                          frame True {
                            n2521 = Bundle(cluster=w4577, "amps"=w4581, "volts"=w4580, "pf"=w4579) -> (w4578:cluster{"amps":dbl, "volts":dbl, "pf":dbl})
                            n2522 = local write "ON L04-2"(w4578) -> ()
                          }
                        }
                      }
                      frame #1 {
                        n2523 = Unbundle(w4586) -> ("amps"=w4585:dbl, "volts"=w4584:dbl, "pf"=w4583:dbl)
                        n2524 = case shown="True" w4587 {
                          tunnel: w4594 -> [_ w4626]
                          tunnel: w4593 -> [_ w4633]
                          tunnel: w4592 -> [_ _]
                          tunnel: w4591 -> [_ _]
                          tunnel: w4590 -> [_ w4632]
                          tunnel: w4589 -> [_ w4631]
                          tunnel: w4588 -> [_ w4596]
                          tunnel: w4585 -> [_ w4628]
                          tunnel: w4584 -> [_ w4627]
                          tunnel: w4583 -> [_ w4625]
                          tunnel: w4582 -> [_ w4617]
                          frame False {
                          }
                          frame True {
                            n2525 = local read "TDMS LAB04-2"() -> (w4630:refnum<k34>)
                            n2526 = Build Array(w4627) -> (w4622:dbl[])
                            n2527 = Build Array(w4625) -> (w4621:dbl[])
                            n2528 = Build Array(w4632) -> (w4620:dbl[])
                            n2529 = Build Array(w4633) -> (w4619:dbl[])
                            n2530 = Build Array(w4628) -> (w4624:dbl[])
